vi "menu-AddMenuGroups.vi"(7 "Menu Name":string[](array[string]), 11 "element":T1[](array[typedef])) -> (3 "Array":T1[](array[typedef]))   [LabVIEW 2017, in "menu-operation.lvlib"]
uses:
  menu-operation.lvlib
  <resource>/Framework/Providers/API/mxLvMenuItem.ctl
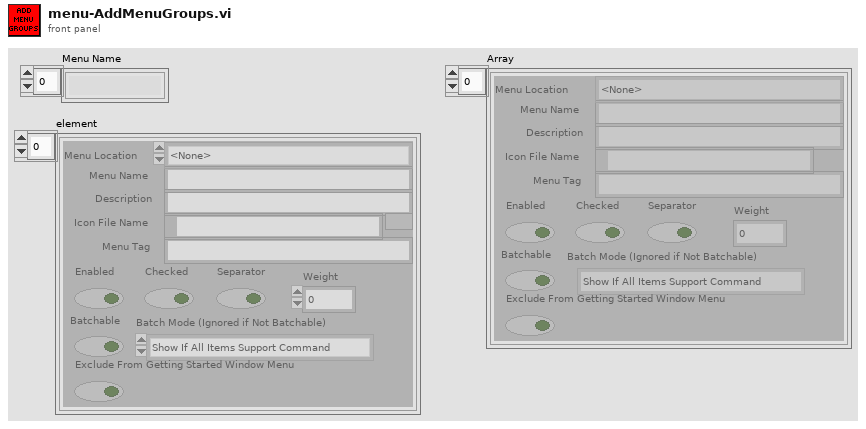
[diagram p1: front panel]
types:
  T1 = typedef "mxLvMenuItem.ctl" = cluster{"Menu Name":string, "Description":string, "Icon File Name":path, "Menu Tag":string, "Enabled":bool, "Checked":bool, "Separator":bool, "Batchable":bool, "Weight":i32, "Batch Mode (Ignored if Not Batchable)":enum32{"Show If All Items Support Command", "Show If Any Items Support Command"}, "Menu Location":enum32{"<None>", "Project", "Project / Build Specifications", "Tools", "Tools / Source Control", "Tools / Real-Time Module", "Help"}, "Exclude From Getting Started Window Menu":bool}
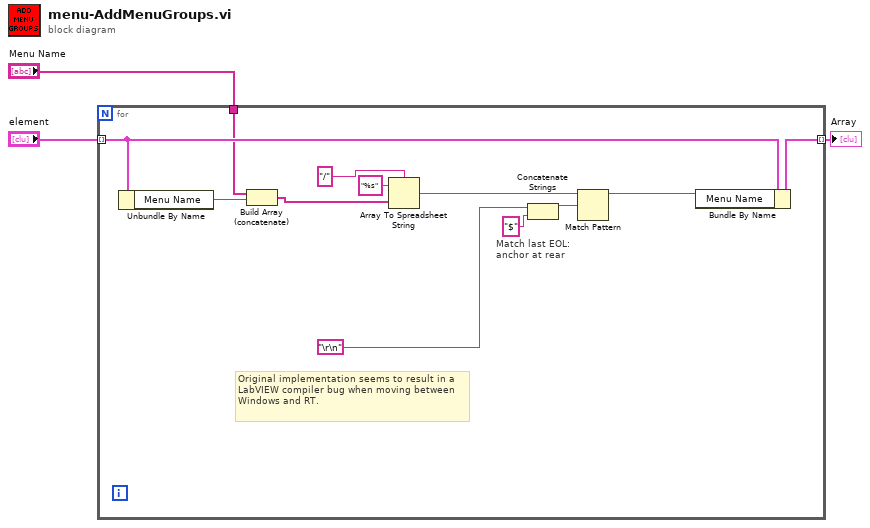
[diagram p0: block diagram]
diagram:
  n1 = for {
    tunnel: "element" -> [w14] mode=indexing
    tunnel: [w15] -> w2 mode=indexing
    tunnel: "Menu Name" -> [w12]
    # "Original implementation seems to result in a LabVIEW compiler bug when moving between Windows and RT."
    # "Match last EOL:\nanchor at rear"
    n2 = Unbundle By Name(w14) -> ("Menu Name"=w9:string)
    n3 = Build Array (concatenate)(w12, w9) -> (w13:string[])
    n4 = Array To Spreadsheet String(delimiter (Tab)="/", array=w13, 3:"%s" ("format string")) -> (spreadsheet string=w7:string)
    n5 = Concatenate Strings("\r\n", "$" ("Substring")) -> (w6:string)
    n6 = Match Pattern(string=w7, regular expression=w6) -> (before substring=w11:string)  [unwired: 1 in, 3 out]
    n7 = Bundle By Name(cluster=w14, "Menu Name"=w11) -> (w15:T1)
  }
  "Array" <- w2
